vi "pointDensity.vi"(8 "Density":ext=0.10000000000000003, 9 "Pen in":bool[](array[boolean]), 10 "Y in":ext[](array[numeric])=[0.0, 0.0, 500.0, 50.0], 11 "X in":ext[](array[numeric])=[500.0, 0.0, 0.0, 250.0]) -> (1 "Pen out":bool[](array[boolean]), 2 "Y out":ext[](array[numeric]), 3 "X out":ext[](array[numeric]))   [LabVIEW 2014]
doc: "André Romero - 2016\nandretec@ifsc.usp.br\n\nIncrease density points of the vector"
panel:
  out "XY Graph Out":cluster{ext[], ext[]}(graph)
  out "XY Graph In":cluster{"Array 5":ext[], "Array 6":ext[]}(graph)={"Array 5"=[500.0, 0.0, 0.0, 250.0], "Array 6"=[0.0, 0.0, 500.0, 50.0]}
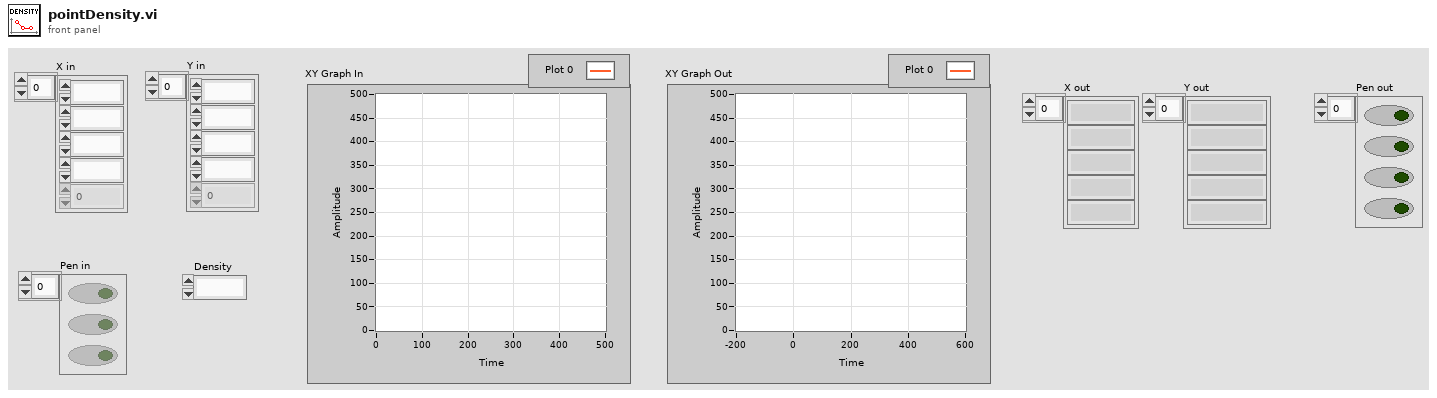
[diagram p1: front panel]
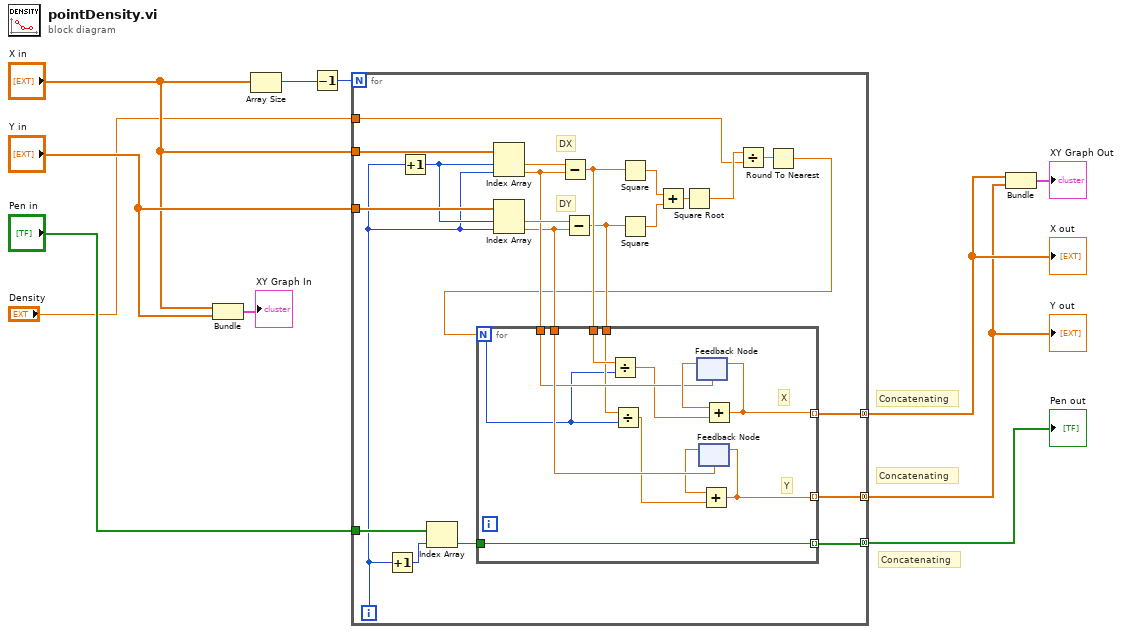
[diagram p0: block diagram]
diagram:
  # "Concatenating"
  # "Concatenating"
  # "Concatenating"
  n1 = Bundle("X in"="X in", "Y in"="Y in") -> (→"XY Graph In":cluster{"X in":ext[], "Y in":ext[]})  [unwired: 1 in]
  n2 = Array Size(array="X in") -> (size(s)=w10:i32)
  n3 = Decrement(x=w10) -> (x-1=w8:i32)
  n4 = for {
    N: w8 -> [_]
    tunnel: "X in" -> [w34]
    tunnel: "Y in" -> [w33]
    tunnel: "Pen in" -> [w25]
    tunnel: "Density" -> [w16]
    tunnel: [w14] -> w3 mode=concatenating
    tunnel: [w13] -> w2 mode=concatenating
    tunnel: [w12] -> w4 mode=concatenating
    i -> [w19]
    # "DY"
    # "DX"
    n5 = Increment(x=w19) -> (x+1=w24:i32)
    n6 = Increment(x=w19) -> (x+1=w20:i32)
    n7 = Index Array(array=w25, index=w24) -> (element=w26:bool)
    n8 = Index Array(array=w34, index #1=w20, index #2=w19) -> (element #1=w28:ext, element #2=w18:ext)
    n9 = Index Array(array=w33, index #1=w20, index #2=w19) -> (element #1=w27:ext, element #2=w17:ext)
    n10 = Subtract(x=w28, y=w18) -> (x-y=w23:ext)
    n11 = Subtract(x=w27, y=w17) -> (x-y=w22:ext)
    n12 = Square(x=w23) -> (x^2=w32:ext)
    n13 = Square(x=w22) -> (x^2=w31:ext)
    n14 = Add(x=w32, y=w31) -> (x+y=w30:ext)
    n15 = Square Root(x=w30) -> (sqrt(x)=w21:ext)
    n16 = Divide(x=w21, y=w16) -> (x/y=w29:ext)
    n17 = Round To Nearest(number=w29) -> (nearest integer value=w15:ext)
    n18 = for {
      N: w15 -> [w37]
      tunnel: w18 -> [w42]
      tunnel: w17 -> [w45]
      tunnel: w23 -> [w39]
      tunnel: w22 -> [w38]
      tunnel: w26 -> [w46]
      tunnel: [w46] -> w12 mode=indexing
      tunnel: [w36] -> w14 mode=indexing
      tunnel: [w35] -> w13 mode=indexing
      # "Y"
      # "X"
      n19 = Divide(x=w39, y=w37) -> (x/y=w41:ext)
      n20 = Divide(x=w38, y=w37) -> (x/y=w40:ext)
      n21 = feedback #1(w42) -> (w44:ext)
      n22 = feedback #2(w45) -> (w43:ext)
      n23 = Add(x=w43, y=w40) -> (x+y=w35:ext)
      n24 = feedback-in #2(w35) -> ()
      n25 = Add(x=w44, y=w41) -> (x+y=w36:ext)
      n26 = feedback-in #1(w36) -> ()
    }
  }
  "X out" <- w3
  "Y out" <- w2
  "Pen out" <- w4
  n27 = Bundle(w3, w2) -> (→"XY Graph Out":cluster{ext[], ext[]})  [unwired: 1 in]
